vi "getReferencePositions.vi"(0 "connection ID":refnum<k5>, 5 "error":errorcluster) -> (14 "connection ID out":refnum<k5>, 15 "position0":dbl, 16 "position1":dbl, 17 "position2":dbl, 19 "error out":errorcluster)   [LabVIEW 2016, in "sen_api.lvlib"]
doc: "Reads out the reference position value of all three measurement axes."
uses:
  sen_api.lvlib
panel:
  out "jsonRespIn":string
  out "JSON-response":string="{\"jsonrpc\":\"2.0\",\"method\":\"\",\"params\":[5,1.245,true,\"name\"],\"id\":\"1\"}"
  out "JSON request":string
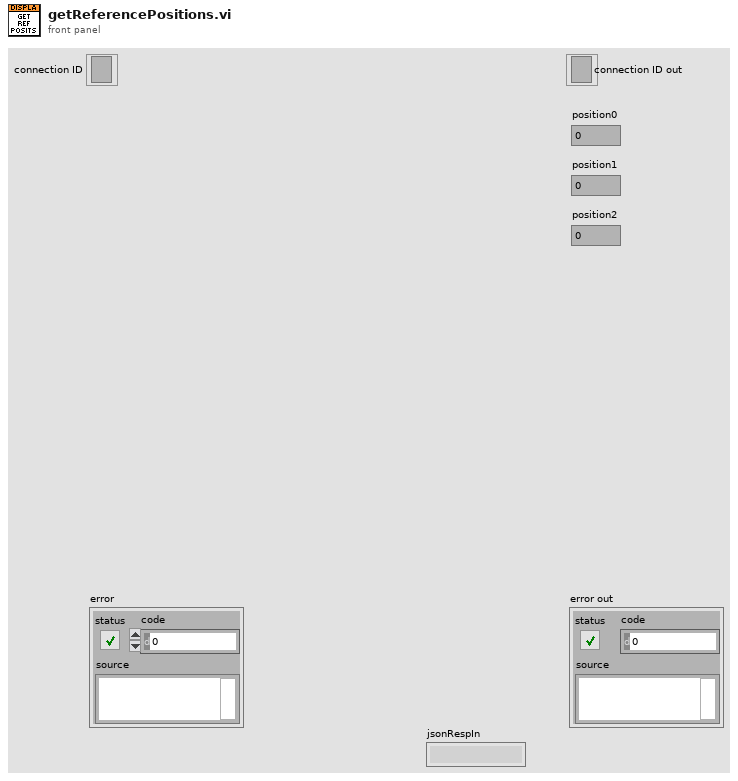
[diagram p1: front panel]
types:
  T1 = cluster{"jsonrpc":string, "method":string, "params":string[], "id":string, "api":i32, "pid":string}
  T2 = enum16{"Standard", "Buffered", "CRLF", "Immediate"}
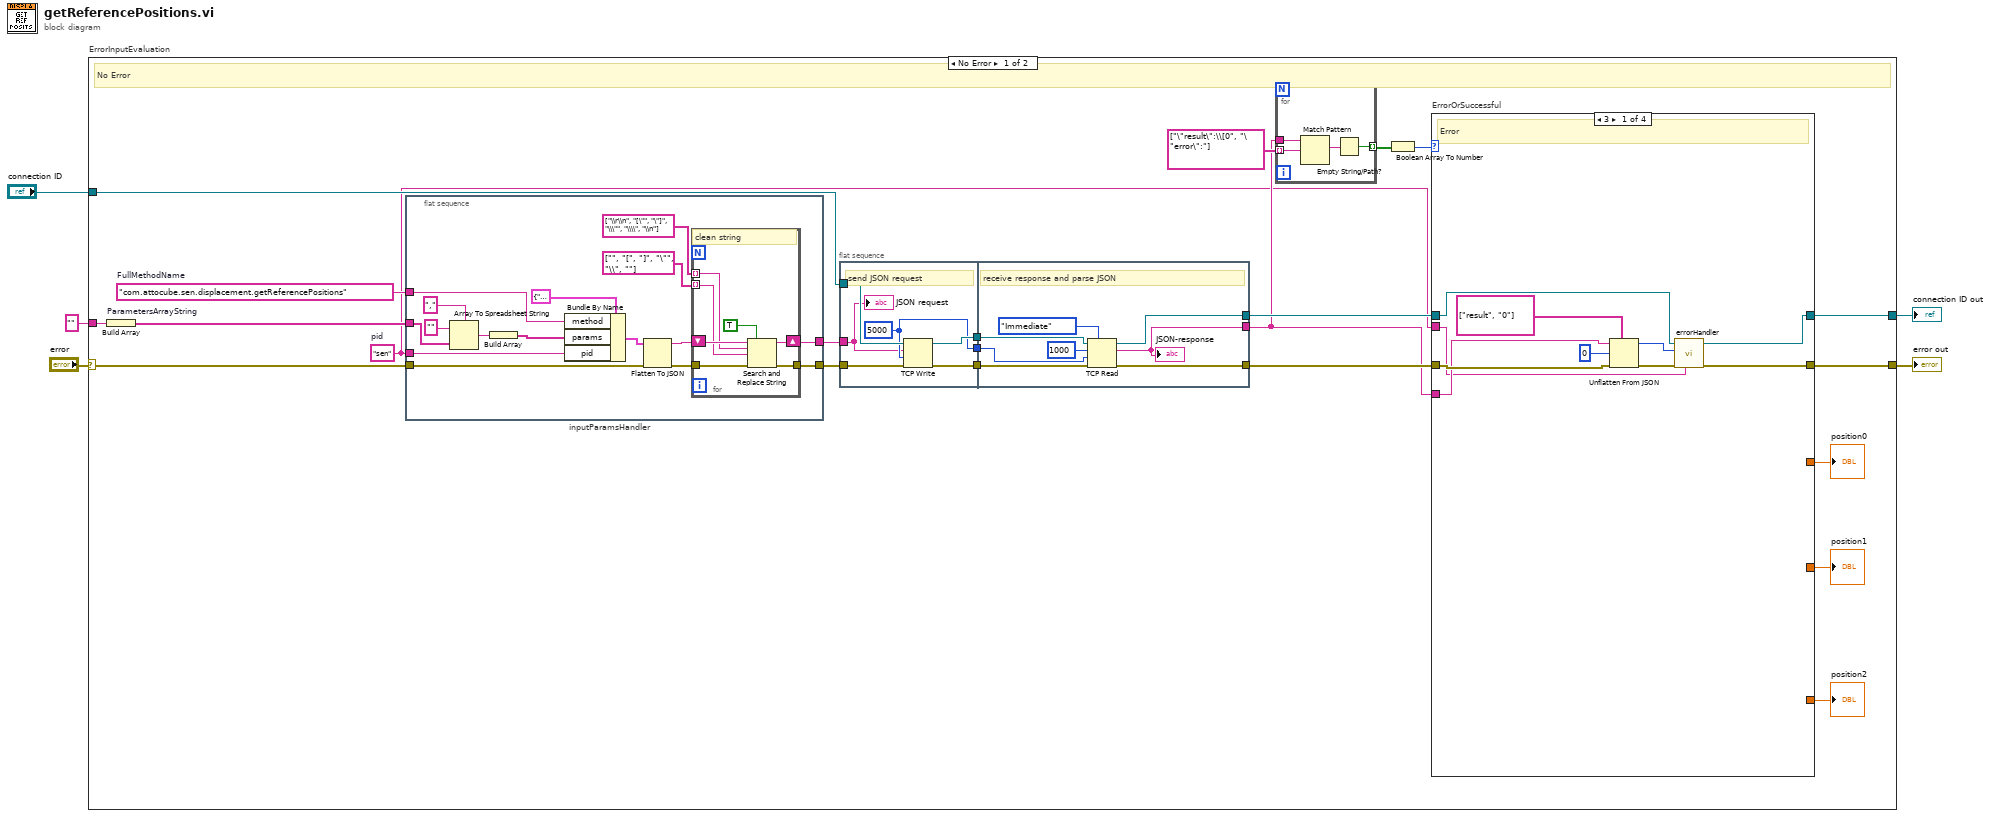
[diagram p0: block diagram]
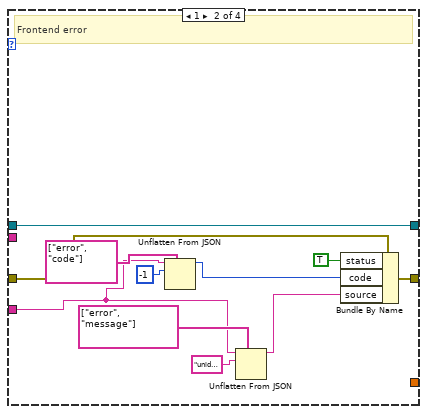
[diagram p2: hidden frame]
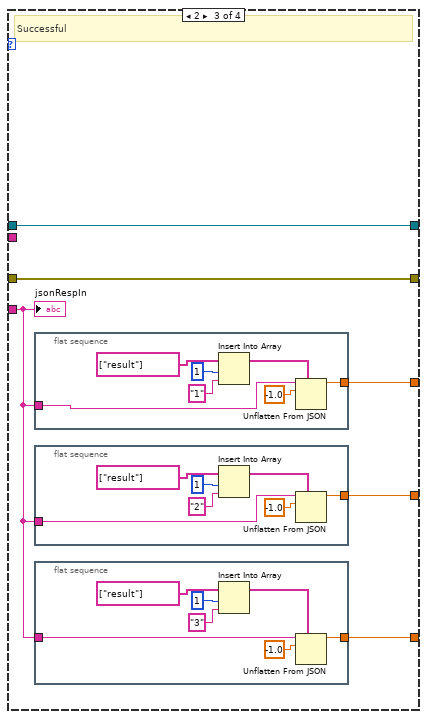
[diagram p3: hidden frame]
diagram:
  n1 = case "ErrorInputEvaluation" shown="No Error" "error" {
    selector: "error" -> [w20 w119]
    tunnel: "connection ID" -> [w24 w120]
    tunnel: [w11 w119] -> w4
    tunnel: [w12 w120] -> w3
    tunnel: "" -> [w9 _]
    frame No Error {
      w10 = "sen"  # pid
      w21 = "com.attocube.sen.displacement.getReferencePositions"  # FullMethodName
      # "No Error"
      n2 = Build Array "ParametersArrayString"(w9) -> (w19:string[])
      n3 = flat-sequence "inputParamsHandler" {
        tunnel: [w81] -> w18
        tunnel: w19 -> [w88]
        tunnel: w20 -> [w86]
        tunnel: [w83] -> w17
        tunnel: w21 -> [w89]
        tunnel: w10 -> [w78]
        frame #0 {
          n4 = Array To Spreadsheet String(delimiter (Tab)=",", array=w88, 3:"" ("format string")) -> (spreadsheet string=w91:string)
          n5 = Build Array "Build Array"(w91) -> (w87:string[])
          n6 = Bundle By Name(cluster=T1 {"jsonrpc"="2.0", "method"="com.attocube.amc.res.setRESReadOutFreq", "params"=[], "id"="1", "api"=2, "pid"=""} ("Cluster"), "method"=w89, "params"=w87, "pid"=w78) -> (w90:T1)
          n7 = Flatten To JSON(anything=w90, error in (no error)=w86) -> (JSON string=w82:string, 11:w84:errorcluster)  [unwired: 1 in]
          n8 = for {
            tunnel: string[] ["\\r\\n", "[\"", "\"]", "\\\"", "\\\\", "\\n"] ("search string") -> [w97] mode=indexing
            tunnel: string[] ["", "[", "]", "\"", "\\", ""] ("replace string (\"\")") -> [w96] mode=indexing
            shift-right: [w99] -> w81
            shift-left: w82 -> [w98]
            tunnel: w84 -> [w95]
            tunnel: [w94] -> w83
            # "clean string"
            n9 = Search and Replace String(replace all?=TRUE ("replace all? (F)"), input string=w98, search string=w97, replace string=w96, error in=w95) -> (result string=w99:string, error out=w94:errorcluster)  [unwired: 3 in, 2 out]
          }
        }
      }
      n10 = flat-sequence {
        tunnel: w24 -> [w110]
        tunnel: [w108] -> w27
        tunnel: [w109] -> w26
        tunnel: w17 -> [w105]
        tunnel: [w107] -> w25
        tunnel: w18 -> [w106]
        tunnel: [w114] -> w16
        tunnel: w27 -> [w116]
        tunnel: w26 -> [w115]
        tunnel: [w112] -> w15
        tunnel: w25 -> [w113]
        tunnel: [w111] -> w14
        frame #0 {
          w107 = 5000 ("timeout ms (25000)")
          # "send JSON request"
          n11 = TCP Write(connection ID=w110, data in=w106, error in (no error)=w105, 9:w107) -> (connection ID out=w108:refnum<k5>, error out=w109:errorcluster)  [unwired: 1 out]
          "JSON request" <- w106
        }
        frame #1 {
          # "receive response and parse JSON"
          n12 = TCP Read(connection ID=w116, bytes to read=1000, error in (no error)=w115, 7:T2."Immediate" ("mode (standard)"), 9:w113) -> (connection ID out=w114:refnum<k5>, data out=w111:string, error out=w112:errorcluster)
          "JSON-response" <- w111
        }
      }
      n13 = for {
        tunnel: string[] ["\"result\":\\[0", "\"error\":"] ("path") -> [w103] mode=indexing
        tunnel: [w101] -> w22 mode=indexing
        tunnel: w14 -> [w104]
        n14 = Match Pattern(string=w104, regular expression=w103) -> (match substring=w102:string)  [unwired: 1 in, 3 out]
        n15 = Empty String/Path?(string/path=w102) -> (empty?=w101:bool)
      }
      n16 = Boolean Array To Number(Boolean array=w22) -> (number=w13:u32)
      n17 = case "ErrorOrSuccessful" shown="3" w13 {
        tunnel: w14 -> [w31 w40 w52 _]
        tunnel: w16 -> [w35 w38 w54 w77]
        tunnel: [w33 w38 w54 w77] -> w12
        tunnel: [w34 w41 w53 w76] -> w11
        tunnel: w15 -> [w37 w39 w53 w76]
        tunnel: w10 -> [w28 _ _ _]
        tunnel: [_ _ w51 _] -> w8
        tunnel: [_ _ w50 _] -> w7
        tunnel: [_ _ w49 _] -> w6
        frame 3 {
          # "Error"
          n18 = Unflatten From JSON(path=string[] ["result", "0"], JSON string=w31, type and defaults=0, error in (no error)=w37) -> (value=w29:i32, error out=w36:errorcluster)  [unwired: 3 in]
          n19 = call "errorHandler.vi"("pid"=w28, "error in"=w36, "errNbr"=w29, "connection ID"=w35) -> ("error out 2"=w34:errorcluster, "connection ID out"=w33:refnum<k5>)  [unwired: 6 in]
        }
        frame 1 {
          # "Frontend error"
          n20 = Unflatten From JSON(path=string[] ["error", "code"], JSON string=w40, type and defaults=-1) -> (value=w47:i32)  [unwired: 4 in, 1 out]
          n21 = Unflatten From JSON(path=string[] ["error", "message"], JSON string=w40, type and defaults="unidentified error") -> (value=w48:string)  [unwired: 4 in, 1 out]
          n22 = Bundle By Name(cluster=w39, "status"=TRUE, "code"=w47, "source"=w48) -> (w41:errorcluster)
        }
        frame 2 {
          # "Successful"
          n23 = flat-sequence "out_double" {
            tunnel: [w69] -> w51
            tunnel: w52 -> [w71]
            frame #0 {
              n24 = Insert Into Array(array=string[] ["result"] ("path"), index=1, new element="1" ("idx")) -> (w73:string[])
              n25 = Unflatten From JSON(path=w73, JSON string=w71, type and defaults=-1.0 ("index")) -> (value=w69:dbl)  [unwired: 4 in, 1 out]
            }
          }
          n26 = flat-sequence "out_double" {
            tunnel: [w62] -> w50
            tunnel: w52 -> [w64]
            frame #0 {
              n27 = Insert Into Array(array=string[] ["result"] ("path"), index=1, new element="2" ("idx")) -> (w66:string[])
              n28 = Unflatten From JSON(path=w66, JSON string=w64, type and defaults=-1.0 ("index")) -> (value=w62:dbl)  [unwired: 4 in, 1 out]
            }
          }
          n29 = flat-sequence "out_double" {
            tunnel: [w55] -> w49
            tunnel: w52 -> [w57]
            frame #0 {
              n30 = Insert Into Array(array=string[] ["result"] ("path"), index=1, new element="3" ("idx")) -> (w59:string[])
              n31 = Unflatten From JSON(path=w59, JSON string=w57, type and defaults=-1.0 ("index")) -> (value=w55:dbl)  [unwired: 4 in, 1 out]
            }
          }
          "jsonRespIn" <- w52
        }
        frame Default {
          # "NoResponse"
        }
      }
      "position0" <- w8
      "position1" <- w7
      "position2" <- w6
    }
    frame Error {
      # "Error"
    }
  }
  "error out" <- w4
  "connection ID out" <- w3
